vi "Vision 대회용.vi"() -> ()   [LabVIEW 2016]
uses:
  <vilib>/vision/Classification.llb/IMAQ Classifier Nearest Neighbor options.ctl
  <vilib>/ptbypt/NI_PtbyPt.lvlib
  <vilib>/vision/NI_Vision_Development_Module.lvlib
panel:
  out "유턴 횟수":u8
  out "정적 횟수":u8
  out "동적 횟수":u8
  out "숫자형":u32
  out "주차점 인식":dbl[](array[numeric])
  in  "탭 컨트롤 2":enum32{"페이지 1", "페이지 2", "페이지 3"}(tab)
  in  "File Path":path=path "C:/Users/SeongHyeon/Desktop/전체프로그램(수정후)(도착후)/Sub Vi/Sensor/Vision Reference/유턴.clf"
  in  "File Path 2":path=path "C:/Users/SeongHyeon/Desktop/전체프로그램(대회당일/Sub Vi/Sensor/Vision Reference/주차.clf"
  in  "File Path 3":path=path "C:/Users/SeongHyeon/Desktop/전체프로그램(대회당일/Sub Vi/Sensor/Vision Reference/동적 장애물 Dark.clf"
  in  "탭 컨트롤":enum32{"유턴", "주차", "동적"}(tab)
  in  "유턴 3":T2={"Preprocessing Options"={"Method"=-1, "Looking for"=1, "Threshold Range"={"Lower value"=0.0, "Upper value"=22.0}, "Threshold Limits"={"Lower value"=0.0, "Upper value"=0.0}, "Reject Border"=FALSE, "# of Erosions"=0, "Kernel Size"={"Lower value"=0, "Upper value"=0}, "Deviation Factor"=0.0}, "Nearest Neighbor Options"={"Method"=0, "Metric"=0, "k"=0}, "Particle Options"={"Scale Dependant"=FALSE, "Scale Factor"=0.0, "Symmetry Dependant"=FALSE, "Symmetry Factor"=0.0}} {"Preprocessing Options"."Deviation Factor" min=0.0; "Preprocessing Options"."Threshold Limits"."Upper value" format="%.2f"; "Preprocessing Options"."Threshold Limits"."Lower value" format="%.2f"; "Preprocessing Options"."Threshold Range"."Upper value" format="%.2f"; "Preprocessing Options"."Threshold Range"."Lower value" format="%.2f"; "Preprocessing Options"."# of Erosions" min=0; "Preprocessing Options"."Method" items=["Manual Threshold"=-1, "-"=-2, "Auto Threshold: Clustering"=0, "Auto Threshold: Entropy"=1, "Auto Threshold: Metric"=2, "Auto Threshold: Moments"=3, "Auto Threshold: Inter-class Variance"=4, "--"=-3, "Local Threshold: Niblack"=5, "Local Threshold: BG Correction"=6]; "Preprocessing Options"."Looking for" items=["Bright Objects", "Dark Objects"]; "Nearest Neighbor Options"."Method" items=["Nearest Neighbor", "K Nearest Neighbor", "Minimum Mean Distance"]; "Nearest Neighbor Options"."Metric" items=["Maximum", "Sum", "Euclidean"]; "Nearest Neighbor Options"."k" min=3}
  in  "주차  3":T2={"Preprocessing Options"={"Method"=-1, "Looking for"=1, "Threshold Range"={"Lower value"=0.0, "Upper value"=26.0}, "Threshold Limits"={"Lower value"=0.0, "Upper value"=0.0}, "Reject Border"=FALSE, "# of Erosions"=0, "Kernel Size"={"Lower value"=0, "Upper value"=0}, "Deviation Factor"=0.0}, "Nearest Neighbor Options"={"Method"=0, "Metric"=0, "k"=0}, "Particle Options"={"Scale Dependant"=FALSE, "Scale Factor"=0.0, "Symmetry Dependant"=FALSE, "Symmetry Factor"=0.0}} {"Preprocessing Options"."Deviation Factor" min=0.0; "Preprocessing Options"."Threshold Limits"."Upper value" format="%.2f"; "Preprocessing Options"."Threshold Limits"."Lower value" format="%.2f"; "Preprocessing Options"."Threshold Range"."Upper value" format="%.2f"; "Preprocessing Options"."Threshold Range"."Lower value" format="%.2f"; "Preprocessing Options"."# of Erosions" min=0; "Preprocessing Options"."Method" items=["Manual Threshold"=-1, "-"=-2, "Auto Threshold: Clustering"=0, "Auto Threshold: Entropy"=1, "Auto Threshold: Metric"=2, "Auto Threshold: Moments"=3, "Auto Threshold: Inter-class Variance"=4, "--"=-3, "Local Threshold: Niblack"=5, "Local Threshold: BG Correction"=6]; "Preprocessing Options"."Looking for" items=["Bright Objects", "Dark Objects"]; "Nearest Neighbor Options"."Method" items=["Nearest Neighbor", "K Nearest Neighbor", "Minimum Mean Distance"]; "Nearest Neighbor Options"."Metric" items=["Maximum", "Sum", "Euclidean"]; "Nearest Neighbor Options"."k" min=3}
  in  "동적 2":T2={"Preprocessing Options"={"Method"=-1, "Looking for"=1, "Threshold Range"={"Lower value"=0.0, "Upper value"=61.0}, "Threshold Limits"={"Lower value"=0.0, "Upper value"=0.0}, "Reject Border"=FALSE, "# of Erosions"=0, "Kernel Size"={"Lower value"=0, "Upper value"=0}, "Deviation Factor"=0.0}, "Nearest Neighbor Options"={"Method"=0, "Metric"=0, "k"=0}, "Particle Options"={"Scale Dependant"=FALSE, "Scale Factor"=0.0, "Symmetry Dependant"=FALSE, "Symmetry Factor"=0.0}} {"Preprocessing Options"."Deviation Factor" min=0.0; "Preprocessing Options"."Threshold Limits"."Upper value" format="%.2f"; "Preprocessing Options"."Threshold Limits"."Lower value" format="%.2f"; "Preprocessing Options"."Threshold Range"."Upper value" format="%.2f"; "Preprocessing Options"."Threshold Range"."Lower value" format="%.2f"; "Preprocessing Options"."# of Erosions" min=0; "Preprocessing Options"."Method" items=["Manual Threshold"=-1, "-"=-2, "Auto Threshold: Clustering"=0, "Auto Threshold: Entropy"=1, "Auto Threshold: Metric"=2, "Auto Threshold: Moments"=3, "Auto Threshold: Inter-class Variance"=4, "--"=-3, "Local Threshold: Niblack"=5, "Local Threshold: BG Correction"=6]; "Preprocessing Options"."Looking for" items=["Bright Objects", "Dark Objects"]; "Nearest Neighbor Options"."Method" items=["Nearest Neighbor", "K Nearest Neighbor", "Minimum Mean Distance"]; "Nearest Neighbor Options"."Metric" items=["Maximum", "Sum", "Euclidean"]; "Nearest Neighbor Options"."k" min=3}
  out "동적":bool
  out "동적":T3 {"Identification Score" format="%.2f"; "Classification Score" format="%.2f"}
  out "주차":bool
  out "Image 2":T4(plugin-control)
  out "출력 클러스터 2":T5
  out "주차 2":T3 {"Identification Score" format="%.2f"; "Classification Score" format="%.2f"}
  in  "Type 2":u32(ring)=3 items=["No Selection", "Point", "Line", "Rectangle", "Oval", "Polygon", "Free", "Annulus", "Unused2", "Unused3", "Broken Line", "Free Hand Line", "Rotated Rectangle"]
  in  "ID 2":enum32{"External", "Internal"}(ring)
  out "유턴":bool
  out "Image":T4(plugin-control)
  out "출력 클러스터":T5
  out "유턴 2":T3 {"Identification Score" format="%.2f"; "Classification Score" format="%.2f"}
  in  "Type":u32(ring)=3 items=["No Selection", "Point", "Line", "Rectangle", "Oval", "Polygon", "Free", "Annulus", "Unused2", "Unused3", "Broken Line", "Free Hand Line", "Rotated Rectangle"]
  in  "ID":enum32{"External", "Internal"}(ring)
  out "횡단보도 거리":dbl[](array[numeric])
  out "헤딩 angle":dbl[][](array[numeric])
  out "Filtered image":T4(plugin-control)
  out "추가된 배열":dbl[][](array[numeric])
  out "프레임 rate":dbl
  out "error out":errorcluster
  in  "Stop (F)":bool
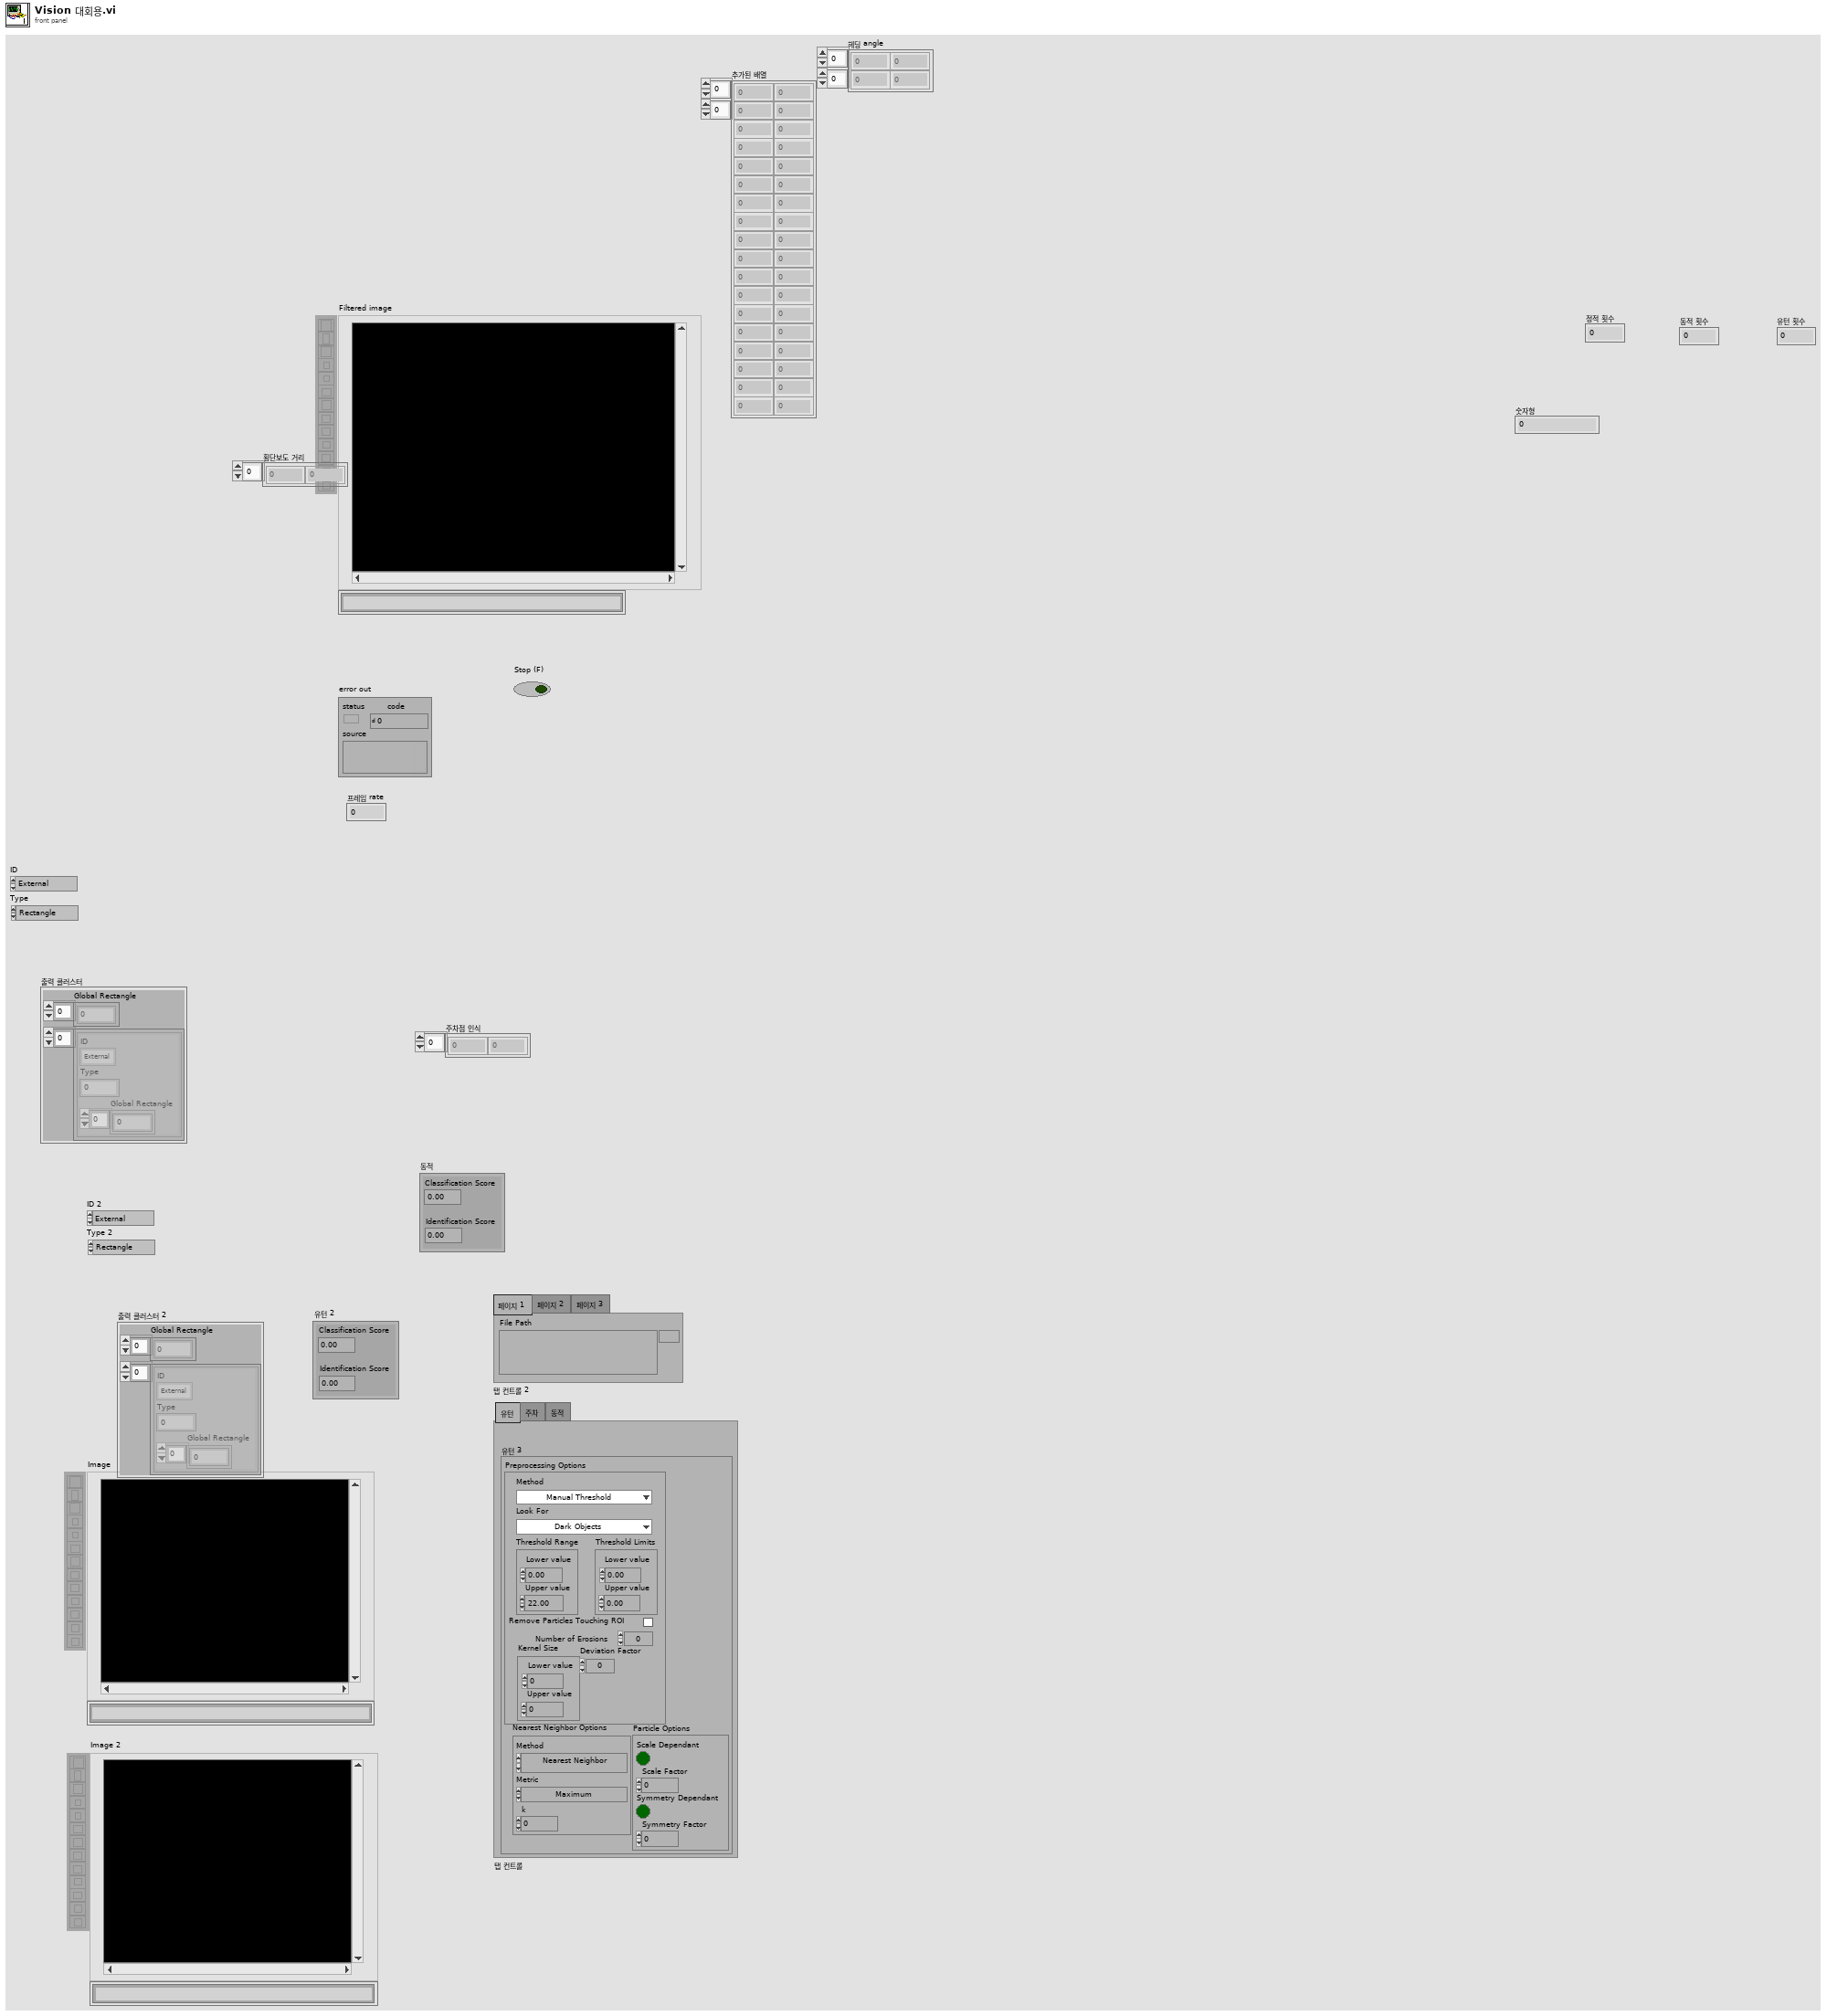
[diagram p1: front panel]
types:
  T1 = typedef "IMAQ Classifier Nearest Neighbor options.ctl" = cluster{"Method":i32, "Metric":i32, "k":i32}
  T2 = cluster{"Preprocessing Options":cluster{"Method":i32, "Looking for":i32, "Threshold Range":cluster{"Lower value":sgl, "Upper value":sgl}, "Threshold Limits":cluster{"Lower value":sgl, "Upper value":sgl}, "Reject Border":bool, "# of Erosions":i32, "Kernel Size":cluster{"Lower value":i32, "Upper value":i32}, "Deviation Factor":dbl}, "Nearest Neighbor Options":T1, "Particle Options":cluster{"Scale Dependant":bool, "Scale Factor":sgl, "Symmetry Dependant":bool, "Symmetry Factor":sgl}}
  T3 = cluster{"Classification Score":sgl, "Identification Score":sgl}
  T4 = typedef "IMAQ Image.ctl" = refnum<image>
  T5 = cluster{"Global Rectangle":i32[], cluster{"ID":enum32{"External", "Internal"}, "Type":u32, "Global Rectangle":i32[]}[]}
  T6 = typedef "Image Type" = u32
  T7 = cluster{"Global Rectangle":cluster{"x1Left":i32, "y1Top":i32, "x2Right":i32, "y2Bottom":i32}, "Centroid":cluster{"x":sgl, "y":sgl}, "Object Size":u32, "Score":dbl}[]
  T8 = cluster{"Position":cluster{"x":sgl, "y":sgl}, "Angle":sgl, "Scale":sgl, "Score":sgl, "Bounding Box":cluster{"x":sgl, "y":sgl}[]}[]
  T9 = cluster{"Position":cluster{"x":sgl, "y":sgl}, "Angle":sgl, "Scale":sgl, "Score":sgl, "Bounding Box":cluster{"x":sgl, "y":sgl}[]}
  T10 = cluster{"Global Rectangle":cluster{"x1Left":i32, "y1Top":i32, "x2Right":i32, "y2Bottom":i32}, "Centroid":cluster{"x":sgl, "y":sgl}, "Object Size":u32, "Score":dbl}
  T11 = cluster{"x1Left":i32, "y1Top":i32, "x2Right":i32, "y2Bottom":i32}
  T12 = cluster{"ID":enum32{"External", "Internal"}, "Type":u32, "Global Rectangle":i32[]}
  T13 = cluster{"ID 2":enum32{"External", "Internal"}, "Type 2":u32, "Global Rectangle":i32[]}
  T14 = cluster{"Calibrated Results (Caliper 1)[0]":sgl, "Calibrated Results (Caliper 1)[1]":sgl, "Calibrated Results (Caliper 1)[2]":sgl, "Calibrated Results (Caliper 1)[3]":sgl, "Calibrated Results (Caliper 1)[4]":sgl, "Calibrated Results (Caliper 1)[5]":sgl, "Calibrated Results (Caliper 1)[6]":sgl, "Calibrated Results (Caliper 1)[7]":sgl, "Calibrated Results (Caliper 1)[8]":sgl}
  T15 = cluster{"Calibrated Results (Caliper 2)[0]":sgl, "Calibrated Results (Caliper 2)[1]":sgl, "Calibrated Results (Caliper 2)[2]":sgl, "Calibrated Results (Caliper 2)[3]":sgl, "Calibrated Results (Caliper 2)[4]":sgl, "Calibrated Results (Caliper 2)[5]":sgl, "Calibrated Results (Caliper 2)[6]":sgl, "Calibrated Results (Caliper 2)[7]":sgl, "Calibrated Results (Caliper 2)[8]":sgl}
  T16 = cluster{"Calibrated Results (Caliper 3)[0]":sgl, "Calibrated Results (Caliper 3)[1]":sgl, "Calibrated Results (Caliper 3)[2]":sgl, "Calibrated Results (Caliper 3)[3]":sgl, "Calibrated Results (Caliper 3)[4]":sgl, "Calibrated Results (Caliper 3)[5]":sgl, "Calibrated Results (Caliper 3)[6]":sgl, "Calibrated Results (Caliper 3)[7]":sgl, "Calibrated Results (Caliper 3)[8]":sgl}
  T17 = cluster{"ID":enum32{"External", "Internal"}, "Type":u32, "Global Rectangle":i32[]}[]
  T18 = cluster{"ID 2":enum32{"External", "Internal"}, "Type 2":u32, "Global Rectangle":i32[]}[]
  T19 = typedef "IMAQ Classifier Session.ctl" = refnum<k1>
  T20 = cluster{"Global Rectangle":i32[], cluster{"ID 2":enum32{"External", "Internal"}, "Type 2":u32, "Global Rectangle":i32[]}[]}
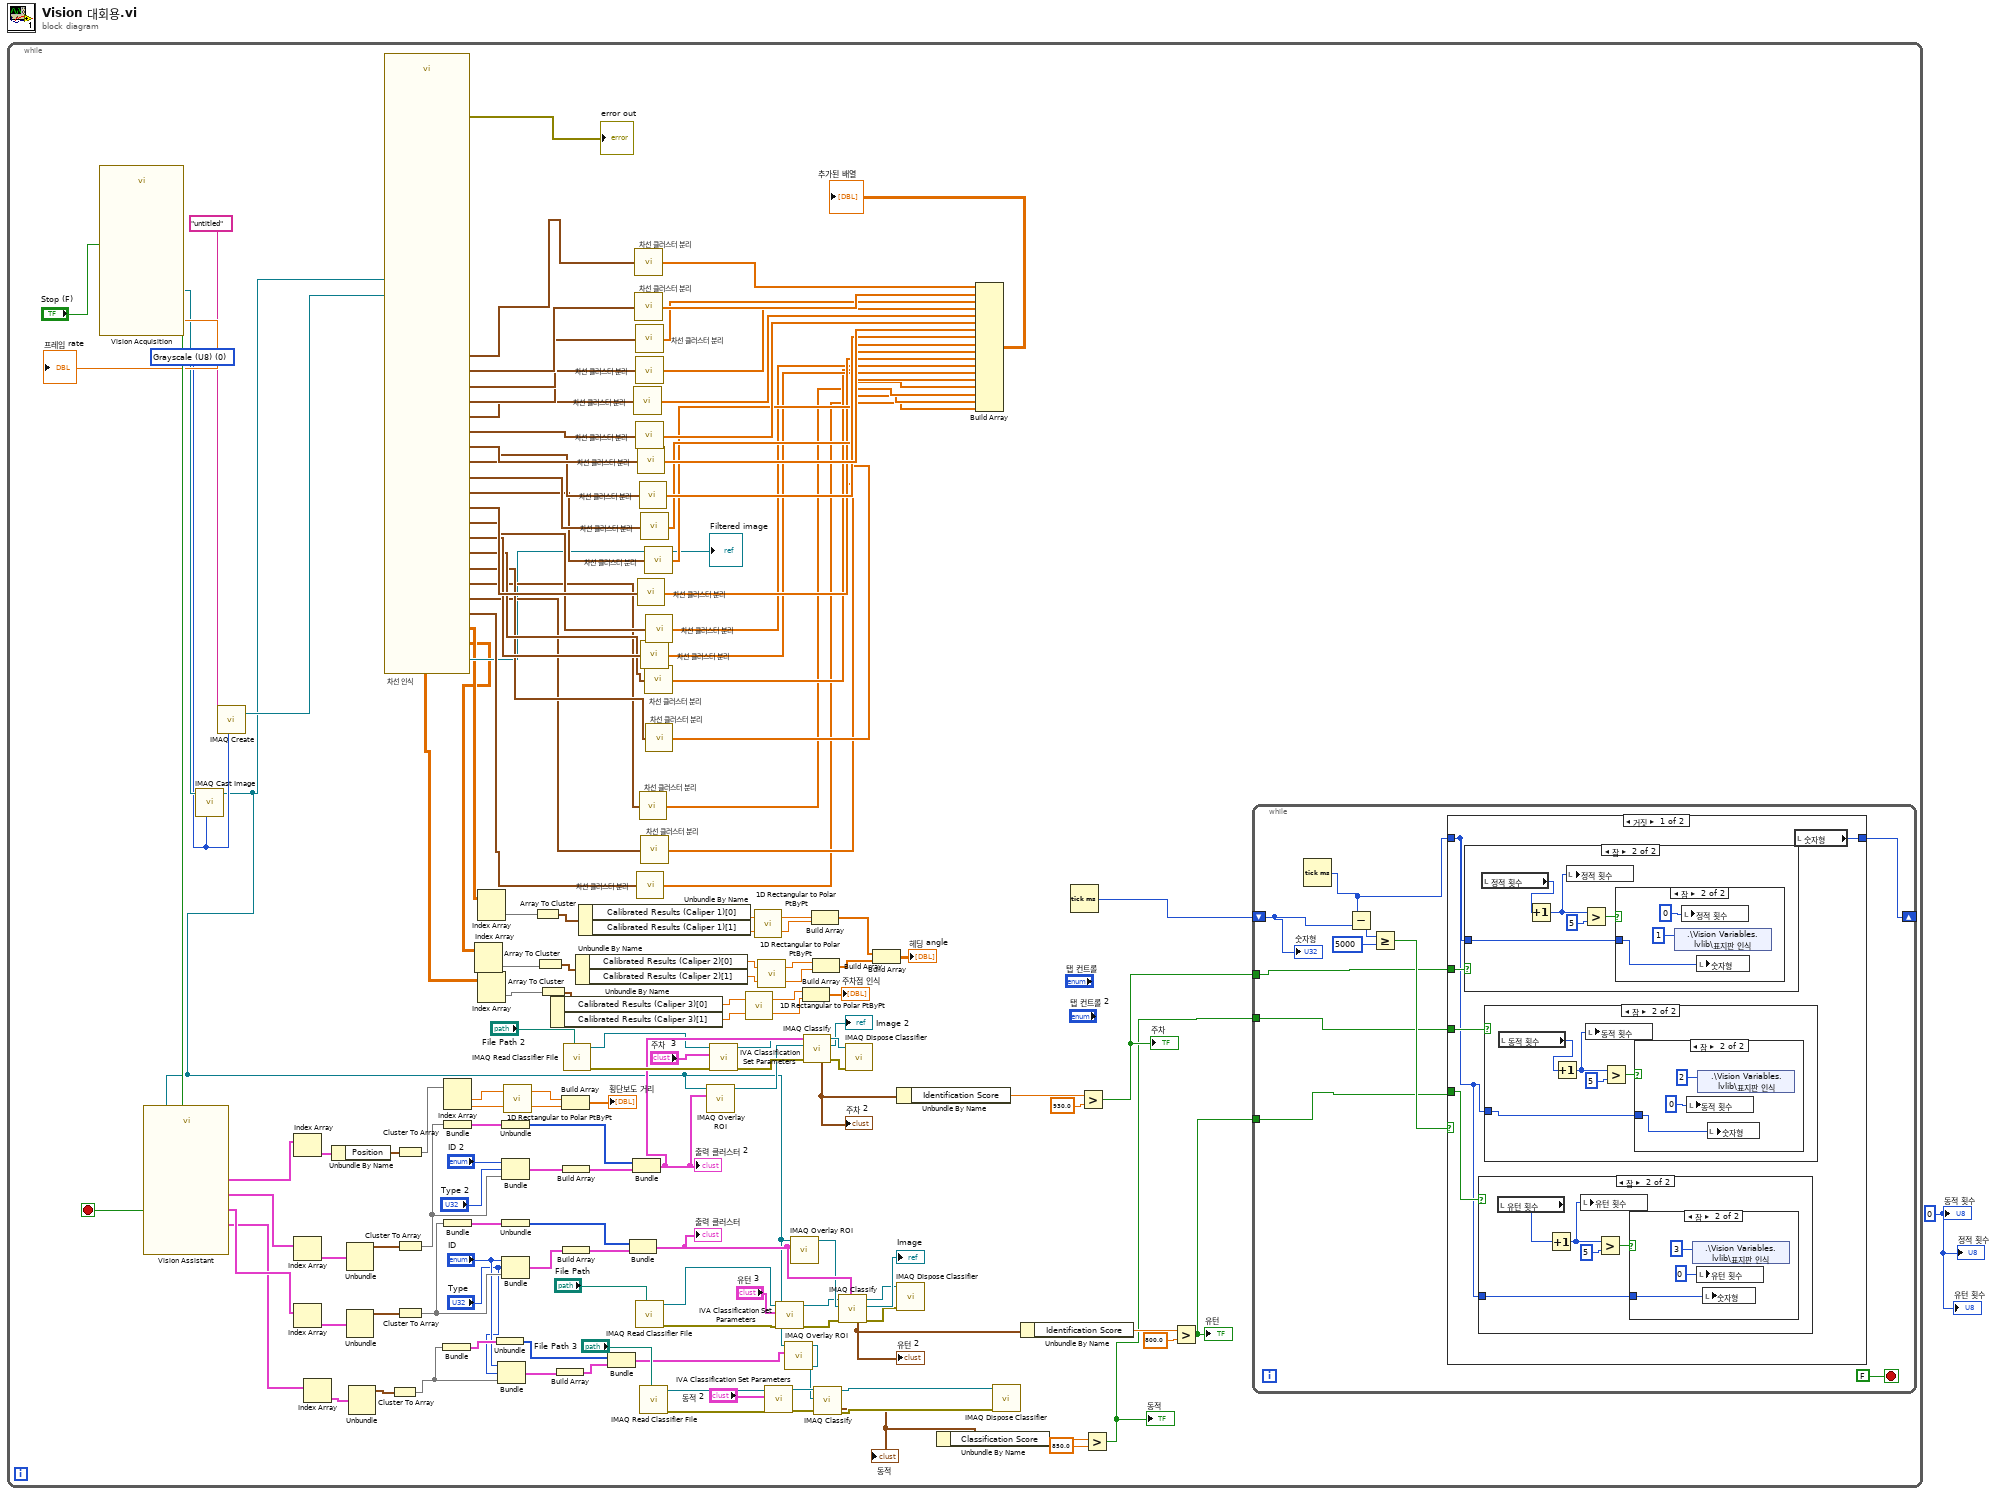
[diagram p0: block diagram]
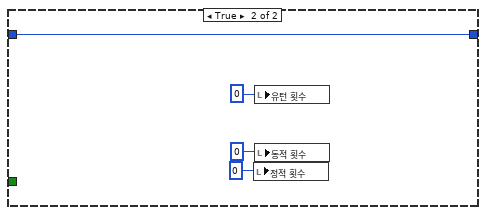
[diagram p8: hidden frame]
diagram:
  w1 = u8 0 ("동적 횟수")
  n1 = while {
    stop <- w154 stop-if-true
    w94 = T6 0 items=["Grayscale (U8)", "Grayscale (I16)", "Grayscale (SGL)", "Complex (CSG)", "RGB (U32)", "HSL (U32)", "RGB (U64)", "Grayscale (U16)"] ("Image Type")
    n2 = call "Vision Acquisition"("Stop (F)"="Stop (F)") -> ("Image Out"=w96:T4, "Frame Rate"=→"프레임 rate":dbl, "Stopped"=w154:bool)  [unwired: 22 in, 2 out]
    n3 = call "IMAQ Cast Image"("Image Type"=w94, "Image Src"=w96) -> ("Image Dst Out"=w18:T4)  [unwired: 8 in, 1 out]
    n4 = call "Vision Assistant"("Image In"=w18) -> ("Shape Report (Shape Matching 3)"=w16:T7, "Shape Report (Shape Matching 2)"=w17:T7, "Calibrated Matches (Pattern Matching 1)"=w84:T8, "Shape Report (Shape Matching 1)"=w15:T7)  [unwired: 21 in, 2 out]
    n5 = call "IMAQ Create"("Image Name"="untitled", "Image Type"=w94) -> ("New Image"=w95:T4)  [unwired: 3 in, 1 out]
    n6 = Index Array(array=w84) -> (element=w92:T9)  [unwired: 1 in]
    n7 = Index Array(array=w17) -> (element=w41:T10)  [unwired: 1 in]
    n8 = Index Array(array=w16) -> (element=w83:T10)  [unwired: 1 in]
    n9 = Index Array(array=w15) -> (element=w39:T10)  [unwired: 1 in]
    n10 = Unbundle By Name(w92) -> ("Position"=w91:cluster{"x":sgl, "y":sgl})
    n11 = Unbundle(w41) -> ("Global Rectangle"=w62:T11)  [unwired: 3 out]
    n12 = Unbundle(w83) -> ("Global Rectangle"=w82:T11)  [unwired: 3 out]
    n13 = Unbundle(w39) -> ("Global Rectangle"=w38:T11)  [unwired: 3 out]
    n14 = call "차선 인식"("Image In"=w18, "Image Dst"=w95) -> ("Calibrated Results (Caliper 3)"=w13:sgl[][], "Calibrated Results (Caliper 1)"=w113:sgl[][], "Edges Coordinates (calibrated) (Edge Detector 21)"=w131:cluster{"X":sgl, "Y":sgl}[], "Edges Coordinates (calibrated) (Edge Detector 20)"=w132:cluster{"X":sgl, "Y":sgl}[], "Edges Coordinates (calibrated) (Edge Detector 19)"=w133:cluster{"X":sgl, "Y":sgl}[], "Edges Coordinates (calibrated) (Edge Detector 18)"=w134:cluster{"X":sgl, "Y":sgl}[], "Calibrated Results (Caliper 2)"=w106:sgl[][], "Edges Coordinates (calibrated) (Edge Detector 17)"=w135:cluster{"X":sgl, "Y":sgl}[], "Edges Coordinates (calibrated) (Edge Detector 16)"=w136:cluster{"X":sgl, "Y":sgl}[], "Edges Coordinates (calibrated) (Edge Detector 15)"=w137:cluster{"X":sgl, "Y":sgl}[], "Edges Coordinates (calibrated) (Edge Detector 13)"=w138:cluster{"X":sgl, "Y":sgl}[], "Edges Coordinates (calibrated) (Edge Detector 12)"=w139:cluster{"X":sgl, "Y":sgl}[], "Edges Coordinates (calibrated) (Edge Detector 11)"=w140:cluster{"X":sgl, "Y":sgl}[], "Edges Coordinates (calibrated) (Edge Detector 10)"=w141:cluster{"X":sgl, "Y":sgl}[], "Edges Coordinates (calibrated) (Edge Detector 8)"=w142:cluster{"X":sgl, "Y":sgl}[], "Edges Coordinates (calibrated) (Edge Detector 7)"=w143:cluster{"X":sgl, "Y":sgl}[], "Edges Coordinates (calibrated) (Edge Detector 5)"=w144:cluster{"X":sgl, "Y":sgl}[], "Image Out"=→"Filtered image":T4, "Edges Coordinates (calibrated) (Edge Detector 1)"=w151:cluster{"X":sgl, "Y":sgl}[], "Edges Coordinates (calibrated) (Edge Detector 2)"=w149:cluster{"X":sgl, "Y":sgl}[], "Edges Coordinates (calibrated) (Edge Detector 3)"=w146:cluster{"X":sgl, "Y":sgl}[], "Edges Coordinates (calibrated) (Edge Detector 4)"=w145:cluster{"X":sgl, "Y":sgl}[], "error out"=→"error out":errorcluster)  [unwired: 1 in, 2 out]
    n15 = Cluster To Array(cluster=w38) -> (array=w37:i32[])
    n16 = Cluster To Array(cluster=w91) -> (array=w90:sgl[])
    n17 = Cluster To Array(cluster=w62) -> (array=w59:i32[])
    n18 = Cluster To Array(cluster=w82) -> (array=w79:i32[])
    n19 = Bundle("Global Rectangle"=w37) -> (w36:cluster{"Global Rectangle":i32[]})  [unwired: 1 in]
    n20 = Index Array(array=w90) -> (element #1=w89:sgl, element #2=w88:sgl)  [unwired: 2 in]
    n21 = Bundle("Global Rectangle"=w59) -> (w61:cluster{"Global Rectangle":i32[]})  [unwired: 1 in]
    n22 = Bundle("Global Rectangle"=w79) -> (w81:cluster{"Global Rectangle":i32[]})  [unwired: 1 in]
    n23 = Index Array(array=w106) -> (element=w105:sgl[])  [unwired: 2 in]
    n24 = Index Array(array=w113) -> (element=w112:sgl[])  [unwired: 2 in]
    n25 = Index Array(array=w13) -> (element=w12:sgl[])  [unwired: 2 in]
    n26 = Unbundle(w36) -> ("Global Rectangle"=w33:i32[])
    n27 = Bundle("ID"="ID", "Type"="Type", "Global Rectangle"=w37) -> (w35:T12)  [unwired: 1 in]
    n28 = Unbundle(w61) -> ("Global Rectangle"=w60:i32[])
    n29 = Bundle("ID 2"="ID 2", "Type 2"="Type 2", "Global Rectangle"=w59) -> (w56:T13)  [unwired: 1 in]
    n30 = Unbundle(w81) -> ("Global Rectangle"=w80:i32[])
    n31 = Bundle("ID"="ID", "Type"="Type", "Global Rectangle"=w79) -> (w78:T12)  [unwired: 1 in]
    n32 = call <vilib>:"1D Rectangular to Polar PtByPt.vi"("y"=w88, "x"=w89) -> ("phase"=w86:dbl, "magnitude"=w87:dbl)
    n33 = Array To Cluster(array=w112) -> (cluster=w111:T14)
    n34 = Array To Cluster(array=w105) -> (cluster=w104:T15)
    n35 = Array To Cluster(array=w12) -> (cluster=w11:T16)
    n36 = Unbundle By Name(w11) -> ("Calibrated Results (Caliper 3)[0]"=w10:sgl, "Calibrated Results (Caliper 3)[1]"=w9:sgl)
    n37 = Build Array(w35) -> (w34:T17)
    n38 = Build Array(w87, w86) -> (→"횡단보도 거리":dbl[])
    n39 = Build Array(w56) -> (w55:T18)
    n40 = Build Array(w78) -> (w77:T17)
    n41 = call "IMAQ Read Classifier File"("File Path"="File Path 2") -> ("error out"=w53:errorcluster, "Classifier Session"=w47:T19)  [unwired: 6 in, 3 out]
    n42 = Unbundle By Name(w104) -> ("Calibrated Results (Caliper 2)[0]"=w103:sgl, "Calibrated Results (Caliper 2)[1]"=w102:sgl)
    n43 = Unbundle By Name(w111) -> ("Calibrated Results (Caliper 1)[0]"=w110:sgl, "Calibrated Results (Caliper 1)[1]"=w109:sgl)
    n44 = Bundle("Global Rectangle"=w33, w34) -> (w26:T5)  [unwired: 1 in]
    n45 = Bundle("Global Rectangle"=w80, w77) -> (w72:T5)  [unwired: 1 in]
    "출력 클러스터" <- w72
    n46 = Bundle("Global Rectangle"=w60, w55) -> (w50:T20)  [unwired: 1 in]
    "출력 클러스터 2" <- w50
    n47 = call "차선 클러스터 분리.vi"("배열"=w144) -> ("R, Theta"=w128:dbl[])
    n48 = call "차선 클러스터 분리.vi"("배열"=w151) -> ("R, Theta"=w150:dbl[])
    n49 = call "차선 클러스터 분리.vi"("배열"=w149) -> ("R, Theta"=w148:dbl[])
    n50 = call "차선 클러스터 분리.vi"("배열"=w146) -> ("R, Theta"=w130:dbl[])
    n51 = call "차선 클러스터 분리.vi"("배열"=w145) -> ("R, Theta"=w129:dbl[])
    n52 = call "차선 클러스터 분리.vi"("배열"=w143) -> ("R, Theta"=w127:dbl[])
    n53 = call "IMAQ Read Classifier File"("File Path"="File Path") -> ("error out"=w75:errorcluster, "Classifier Session"=w68:T19)  [unwired: 6 in, 3 out]
    n54 = call "차선 클러스터 분리.vi"("배열"=w131) -> ("R, Theta"=w114:dbl[])
    n55 = call "차선 클러스터 분리.vi"("배열"=w142) -> ("R, Theta"=w126:dbl[])
    n56 = call "차선 클러스터 분리.vi"("배열"=w138) -> ("R, Theta"=w122:dbl[])
    n57 = call "차선 클러스터 분리.vi"("배열"=w141) -> ("R, Theta"=w125:dbl[])
    n58 = call "차선 클러스터 분리.vi"("배열"=w133) -> ("R, Theta"=w116:dbl[])
    n59 = call "IMAQ Read Classifier File"("File Path"="File Path 3") -> ("error out"=w24:errorcluster, "Classifier Session"=w29:T19)  [unwired: 6 in, 3 out]
    n60 = call "차선 클러스터 분리.vi"("배열"=w140) -> ("R, Theta"=w124:dbl[])
    n61 = call "차선 클러스터 분리.vi"("배열"=w136) -> ("R, Theta"=w120:dbl[])
    n62 = call "차선 클러스터 분리.vi"("배열"=w132) -> ("R, Theta"=w115:dbl[])
    n63 = call "차선 클러스터 분리.vi"("배열"=w139) -> ("R, Theta"=w123:dbl[])
    n64 = call "차선 클러스터 분리.vi"("배열"=w135) -> ("R, Theta"=w119:dbl[])
    n65 = call "차선 클러스터 분리.vi"("배열"=w137) -> ("R, Theta"=w121:dbl[])
    n66 = call "차선 클러스터 분리.vi"("배열"=w134) -> ("R, Theta"=w117:dbl[])
    n67 = call "IMAQ Overlay ROI"("ROI Descriptor"=w50, "Image"=w18) -> ("Image Out"=w49:T4)  [unwired: 8 in, 1 out]
    n68 = call <vilib>:"IVA Classification Set Parameters.vi"("error in"=w53, "Paramaters"="주차  3", "Classifier Session In"=w47) -> ("error out"=w52:errorcluster, "Classifier Session Out"=w48:T19)  [unwired: 7 out]
    n69 = call <vilib>:"1D Rectangular to Polar PtByPt.vi"("y"=w9, "x"=w10) -> ("phase"=w7:dbl, "magnitude"=w8:dbl)
    n70 = call <vilib>:"1D Rectangular to Polar PtByPt.vi"("y"=w109, "x"=w110) -> ("phase"=w107:dbl, "magnitude"=w108:dbl)
    n71 = call <vilib>:"1D Rectangular to Polar PtByPt.vi"("y"=w102, "x"=w103) -> ("phase"=w100:dbl, "magnitude"=w101:dbl)
    n72 = call <vilib>:"IVA Classification Set Parameters.vi"("error in"=w24, "Paramaters"="동적 2", "Classifier Session In"=w29) -> ("error out"=w23:errorcluster, "Classifier Session Out"=w28:T19)  [unwired: 7 out]
    n73 = call <vilib>:"IVA Classification Set Parameters.vi"("error in"=w75, "Paramaters"="유턴 3", "Classifier Session In"=w68) -> ("error out"=w74:errorcluster, "Classifier Session Out"=w69:T19)  [unwired: 7 out]
    n74 = call "IMAQ Overlay ROI"("ROI Descriptor"=w26, "Image"=w18) -> ("Image Out"=w25:T4)  [unwired: 8 in, 1 out]
    n75 = call "IMAQ Overlay ROI"("ROI Descriptor"=w72, "Image"=w18) -> ("Image Out"=w71:T4)  [unwired: 8 in, 1 out]
    n76 = Build Array(w8, w7) -> (→"주차점 인식":dbl[])
    n77 = call "IMAQ Classify"("ROI Descriptor"=w50, "error in (no error)"=w52, "Image"=w49, "Classifier Session"=w48) -> ("error out"=w42:errorcluster, "Image (dup)"=→"Image 2":T4, "Classifier Session (dup)"=w43:T19, "Scores"=w46:T3)  [unwired: 2 in, 2 out]
    "주차 2" <- w46
    n78 = Build Array(w108, w107) -> (w99:dbl[])
    n79 = Build Array(w101, w100) -> (w98:dbl[])
    n80 = call "IMAQ Classify"("error in (no error)"=w23, "Image"=w25, "Classifier Session"=w28) -> ("error out"=w22:errorcluster, "Classifier Session (dup)"=w27:T19, "Scores"=w21:T3)  [unwired: 3 in, 3 out]
    "동적" <- w21
    n81 = call "IMAQ Classify"("ROI Descriptor"=w72, "error in (no error)"=w74, "Image"=w71, "Classifier Session"=w69) -> ("error out"=w63:errorcluster, "Image (dup)"=→"Image":T4, "Classifier Session (dup)"=w64:T19, "Scores"=w67:T3)  [unwired: 2 in, 2 out]
    "유턴 2" <- w67
    n82 = call "IMAQ Dispose Classifier"("error in (no error)"=w42, "Classifier Session"=w43) -> ()  [unwired: 9 in, 1 out]
    n83 = Build Array(w99, w98) -> (→"헤딩 angle":dbl[][])
    n84 = Unbundle By Name(w46) -> ("Identification Score"=w45:sgl)
    n85 = call "IMAQ Dispose Classifier"("error in (no error)"=w63, "Classifier Session"=w64) -> ()  [unwired: 9 in, 1 out]
    n86 = Unbundle By Name(w21) -> ("Classification Score"=w20:sgl)
    n87 = Build Array(w150, w148, w130, w129, w128, w127, w126, w125, w124, w123, w122, w121, w120, w119, w117, w116, w115, w114) -> (→"추가된 배열":dbl[][])
    n88 = call "IMAQ Dispose Classifier"("error in (no error)"=w22, "Classifier Session"=w27) -> ()  [unwired: 9 in, 1 out]
    n89 = Unbundle By Name(w67) -> ("Identification Score"=w66:sgl)
    n90 = Tick Count (ms)() -> (millisecond timer value=w5:u32)
    n91 = Greater?(x=w45, y=sgl 930.0) -> (0:w4:bool)
    "주차" <- w4
    n92 = Greater?(x=w20, y=sgl 850.0) -> (0:w3:bool)
    "동적" <- w3
    n93 = Greater?(x=w66, y=sgl 800.0) -> (0:w2:bool)
    "유턴" <- w2
    n94 = while {
      shift-right: [w160] -> _
      shift-left: w5 -> [w159]
      tunnel: w4 -> [w158]
      tunnel: w3 -> [w157]
      tunnel: w2 -> [w156]
      stop <- FALSE stop-if-true
      n95 = Tick Count (ms)() -> (millisecond timer value=w161:u32)
      n96 = Subtract(x=w161, y=w159) -> (x-y=w164:u32)
      n97 = Greater Or Equal?(x=w164, y=u32 5000 ("x-y")) -> (x >= y?=w162:bool)
      n98 = case shown="거짓" w162 {
        tunnel: w158 -> [w170 _]
        tunnel: w157 -> [w169 _]
        tunnel: w156 -> [w168 _]
        tunnel: w161 -> [w166 w198]
        tunnel: [w167 w198] -> w160
        frame False {
          n99 = case shown="참" w170 {
            tunnel: w166 -> [_ w187]
            frame False {
            }
            frame True {
              n100 = local read "정적 횟수"() -> (w188:u8)
              n101 = Increment(x=w188) -> (x+1=w190:u8)
              n102 = local write "정적 횟수"(w190) -> ()
              n103 = Greater?(x=w190, y=u8 5) -> (0:w189:bool)
              n104 = case shown="참" w189 {
                tunnel: w187 -> [_ w192]
                frame False {
                }
                frame True {
                  n105 = shared-variable ".\\Vision Variables.lvlib\\표지판 인식"(u8 1 ("표지판 인식")) -> ()  [unwired: 1 in, 1 out]
                  n106 = local write "정적 횟수"(u8 0 ("정적 횟수")) -> ()
                  n107 = local write "숫자형"(w192) -> ()
                }
              }
            }
          }
          n108 = case shown="참" w168 {
            tunnel: w166 -> [_ w171]
            frame False {
            }
            frame True {
              n109 = local read "유턴 횟수"() -> (w172:u8)
              n110 = Increment(x=w172) -> (x+1=w174:u8)
              n111 = local write "유턴 횟수"(w174) -> ()
              n112 = Greater?(x=w174, y=u8 5) -> (0:w173:bool)
              n113 = case shown="참" w173 {
                tunnel: w171 -> [_ w176]
                frame False {
                }
                frame True {
                  n114 = shared-variable ".\\Vision Variables.lvlib\\표지판 인식"(u8 3 ("표지판 인식")) -> ()  [unwired: 1 in, 1 out]
                  n115 = local write "유턴 횟수"(u8 0 ("정적 횟수")) -> ()
                  n116 = local write "숫자형"(w176) -> ()
                }
              }
            }
          }
          n117 = case shown="참" w169 {
            tunnel: w166 -> [_ w179]
            frame False {
            }
            frame True {
              n118 = local read "동적 횟수"() -> (w180:u8)
              n119 = Increment(x=w180) -> (x+1=w182:u8)
              n120 = local write "동적 횟수"(w182) -> ()
              n121 = Greater?(x=w182, y=u8 5) -> (0:w181:bool)
              n122 = case shown="참" w181 {
                tunnel: w179 -> [_ w184]
                frame False {
                }
                frame True {
                  n123 = local write "동적 횟수"(u8 0 ("정적 횟수")) -> ()
                  n124 = shared-variable ".\\Vision Variables.lvlib\\표지판 인식"(u8 2 ("표지판 인식")) -> ()  [unwired: 1 in, 1 out]
                  n125 = local write "숫자형"(w184) -> ()
                }
              }
            }
          }
          n126 = local read "숫자형"() -> (w167:u32)
        }
        frame True {
          n127 = local write "정적 횟수"(u8 0 ("정적 횟수")) -> ()
          n128 = local write "유턴 횟수"(u8 0 ("정적 횟수")) -> ()
          n129 = local write "동적 횟수"(u8 0 ("정적 횟수")) -> ()
        }
      }
      "숫자형" <- w159
    }
  }
  "동적 횟수" <- w1
  "정적 횟수" <- w1
  "유턴 횟수" <- w1
